vi "Read Buffer Chan Queue.vi"(8 "error in (no error)":errorcluster, 11 "DataProcessor in":refnum<class "DataProcessor.lvclass">) -> (0 "error out":errorcluster, 2 "Buffer Queue":refnum<queue>, 3 "DataProcessor out":refnum<class "DataProcessor.lvclass">)   [LabVIEW 2010, in "DataProcessor.lvclass"]
uses:
  DataProcessor.lvclass
  DataProcessor.lvclass/DataProcessor.ctl
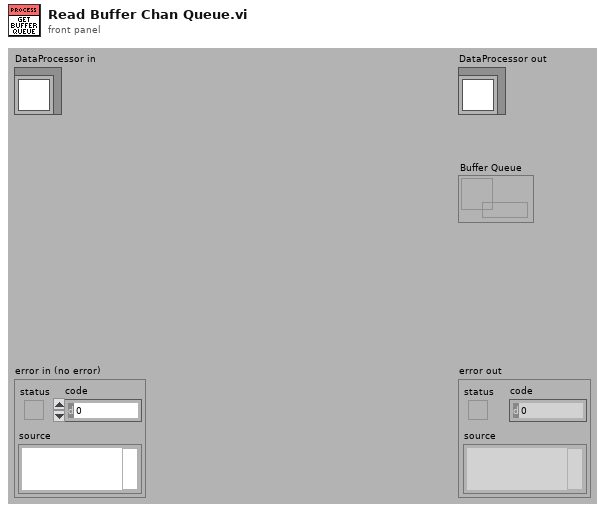
[diagram p1: front panel]
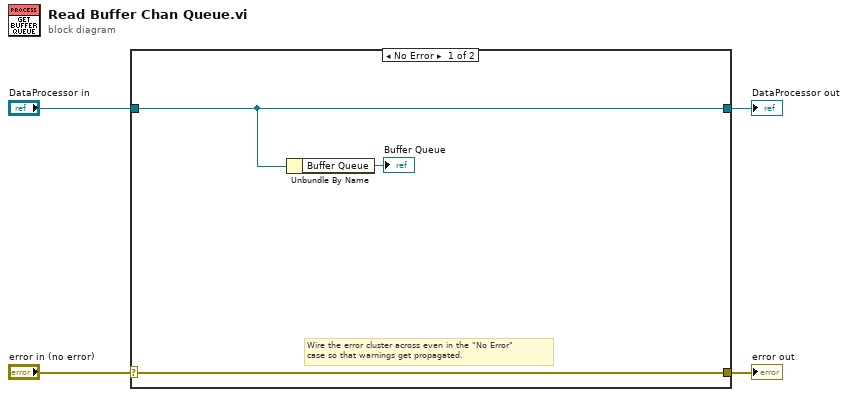
[diagram p0: block diagram]
diagram:
  n1 = case shown="No Error" "error in (no error)" {
    selector: "error in (no error)" -> [w7 w9]
    tunnel: [w7 w9] -> w3
    tunnel: [w6 w8] -> w1
    tunnel: "DataProcessor in" -> [w6 w8]
    frame No Error {
      # "Wire the error cluster across even in the \"No Error\"\ncase so that warnings get propagated."
      n2 = Unbundle By Name(w6) -> ("Buffer Queue"=→"Buffer Queue":refnum<queue>)
    }
    frame Error {
    }
  }
  "error out" <- w3
  "DataProcessor out" <- w1
